vi "Write NS (RT).vi"(8 "error in (no error)":errorcluster, 10 "Message Data":variant, 11 "Message":string) -> (0 "error out":errorcluster)   [LabVIEW 2021]
uses:
  support/Message Queue/Message Cluster.ctl
  Global Variables/Network Globals.vi
  support/Message Queue/Message Queue.lvlib
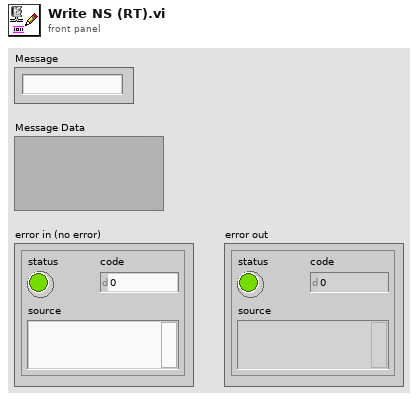
[diagram p1: front panel]
types:
  T1 = typedef "Message Queue.lvlib/Message Cluster.ctl" = cluster{"Message":string, "Message Data":variant}
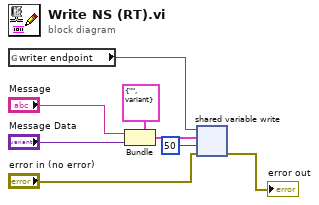
[diagram p0: block diagram]
diagram:
  n1 = global read "Network Globals.vi" "writer endpoint"() -> (w4:refnum<k21>)
  n2 = Bundle(cluster=T1 {"Message"="", "Message Data"=variant} ("Message Cluster"), "Message"="Message", "Message Data"="Message Data") -> (w3:T1)
  n3 = shared-variable-write(w4, "error in (no error)", w3, 50 ("timeout ms (-1)")) -> (→"error out":errorcluster)  [unwired: 2 out]
